vi "Database.Global.vi"() -> ()   [LabVIEW 2016]
uses:
  Database.Main.Data.Sets.ctl
  Database.Main.Data.Status.ctl
panel:
  out "DB.Time.Offset":dbl
  out "DB.Status":T1
  in  "DB.Sets":T2
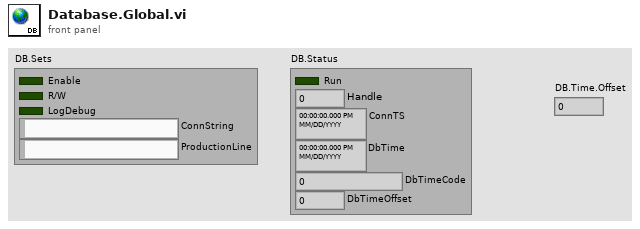
[diagram p1: front panel]
types:
  T1 = typedef "Database.Main.Data.Status.ctl" = cluster{"Run":bool, "Handle":i32, "ConnTS":timestamp, "DbTime":timestamp, "DbTimeCode":dbl, "DbTimeOffset":dbl}
  T2 = typedef "Database.Main.Data.Sets.ctl" = cluster{"Enable":bool, "R/W":bool, "LogDebug":bool, "ConnString":string, "ProductionLine":string}
diagram:
